vi "MNIST_weight print_sub.vi"(1 "최소값":dbl=-255.0, 2 "최대값":dbl=255.0, 3 "배열":dbl[][](array[numeric])=[[-5.0, -1.0, 4.0, -1.0, -5.0, -4.0, -5.0, -5.0, -5.0, -1.0, 4.0, -2.0, -5.0, -4.0, 4.0, 4.0, 5.0, 4.0, 4.0, 2.0, -3.0, -5.0, -1.0, 3.0, 5.0, 5.0, 0.0, 1.0], [-4.0, -5.0, 4.0, 2.0, 3.0, 5.0, -3.0, -5.0, -5.0, -5.0, -5.0, -5.0, -5.0, -5.0, -5.0, -5.0, -5.0, -5.0, -5.0, -5.0, -5.0, -5.0, -5.0, -5.0, -1.0, -5.0, 5.0, -3.0], [0.0, -5.0, -5.0, -5.0, -5.0, -5.0, -5.0, -5.0, -5.0, -5.0, -6.0, -6.0, -6.0, -6.0, -6.0, -6.0, -6.0, -7.0, -6.0, -6.0, -6.0, -6.0, -5.0, -5.0, 4.0, 4.0, -5.0, -2.0], [-2.0, -5.0, 2.0, -5.0, -5.0, -5.0, -5.0, -6.0, -6.0, -6.0, -7.0, -7.0, -7.0, -8.0, -10.0, -10.0, -7.0, -7.0, -9.0, -7.0, -10.0, -8.0, -7.0, -7.0, -6.0, -2.0, 0.0, 0.0], [-5.0, -5.0, 2.0, -5.0, -1.0, -5.0, -6.0, -7.0, -10.0, -15.0, -15.0, -14.0, -14.0, -12.0, -14.0, -26.0, -26.0, -18.0, -18.0, -22.0, -23.0, -19.0, -14.0, -9.0, -7.0, -5.0, -5.0, -5.0], [-5.0, 0.0, 2.0, -5.0, -5.0, -7.0, -7.0, -9.0, -14.0, -28.0, -32.0, -42.0, -44.0, -45.0, -53.0, -58.0, -56.0, -63.0, -53.0, -45.0, -47.0, -42.0, -29.0, -18.0, -10.0, -7.0, -5.0, -5.0], [5.0, -5.0, -5.0, -6.0, -8.0, -7.0, -10.0, -22.0, -30.0, -44.0, -37.0, -25.0, 7.0, 28.0, 51.0, 43.0, 22.0, -1.0, -16.0, -39.0, -51.0, -48.0, -35.0, -17.0, -9.0, -7.0, -6.0, -5.0], [1.0, -5.0, -7.0, -8.0, -8.0, -11.0, -17.0, -29.0, -37.0, -30.0, -3.0, 31.0, 72.0, 92.0, 96.0, 93.0, 86.0, 52.0, 27.0, -12.0, -39.0, -45.0, -29.0, -10.0, -9.0, -7.0, -7.0, -5.0], [-5.0, -6.0, -7.0, -8.0, -10.0, -16.0, -17.0, -23.0, -15.0, -9.0, 24.0, 66.0, 83.0, 55.0, 34.0, 22.0, 45.0, 38.0, 30.0, 5.0, -22.0, -34.0, -31.0, -20.0, -11.0, -8.0, -7.0, -5.0], [-5.0, -6.0, -7.0, -7.0, -14.0, -15.0, -10.0, -8.0, 6.0, 21.0, 62.0, 73.0, 34.0, 4.0, -19.0, -36.0, -5.0, 16.0, 29.0, 24.0, 2.0, -21.0, -31.0, -17.0, -12.0, -8.0, -7.0, -5.0], [-5.0, -6.0, -7.0, -7.0, -16.0, -7.0, 10.0, 21.0, 28.0, 41.0, 56.0, 38.0, 0.0, -25.0, -40.0, -19.0, 13.0, 34.0, 36.0, 35.0, 16.0, -14.0, -19.0, -12.0, -8.0, -7.0, -7.0, -5.0], [-5.0, -6.0, -7.0, -7.0, -11.0, 7.0, 15.0, 42.0, 53.0, 44.0, 35.0, 9.0, -43.0, -46.0, -33.0, -10.0, 35.0, 51.0, 58.0, 60.0, 27.0, 6.0, -14.0, -9.0, -7.0, -6.0, -6.0, -5.0], [-5.0, -6.0, -6.0, -5.0, 7.0, 14.0, 30.0, 59.0, 56.0, 33.0, 14.0, -17.0, -48.0, -42.0, -24.0, 9.0, 35.0, 47.0, 75.0, 74.0, 27.0, -1.0, -12.0, -10.0, -7.0, -7.0, -7.0, -5.0], [-5.0, -5.0, -6.0, -2.0, 7.0, 17.0, 37.0, 64.0, 65.0, 19.0, 10.0, -19.0, -40.0, -18.0, -8.0, 10.0, 44.0, 72.0, 71.0, 43.0, 8.0, -4.0, -17.0, -17.0, -9.0, -7.0, -6.0, -5.0], [-5.0, -5.0, -6.0, 4.0, 3.0, 8.0, 26.0, 58.0, 67.0, 24.0, 7.0, -4.0, -4.0, -10.0, -4.0, 25.0, 60.0, 89.0, 60.0, 5.0, -26.0, -29.0, -21.0, -20.0, -10.0, -6.0, -5.0, -4.0], [-5.0, 5.0, -7.0, -8.0, -5.0, -7.0, 12.0, 39.0, 60.0, 48.0, 45.0, 33.0, 23.0, 3.0, 14.0, 42.0, 75.0, 66.0, 21.0, -21.0, -41.0, -43.0, -25.0, -17.0, -10.0, -6.0, -5.0, -5.0], [-5.0, -5.0, -6.0, -9.0, -9.0, -18.0, -2.0, 18.0, 42.0, 46.0, 55.0, 42.0, 18.0, 7.0, 22.0, 51.0, 65.0, 55.0, -2.0, -25.0, -35.0, -44.0, -18.0, -15.0, -10.0, -7.0, -5.0, -5.0], [-4.0, -5.0, -5.0, -8.0, -15.0, -23.0, -12.0, 1.0, 18.0, 28.0, 44.0, 37.0, 22.0, 13.0, 25.0, 59.0, 58.0, 28.0, 7.0, -21.0, -46.0, -40.0, -24.0, -14.0, -9.0, -6.0, -5.0, -5.0], [5.0, -5.0, -5.0, -7.0, -13.0, -23.0, -25.0, -11.0, -8.0, -9.0, 9.0, 1.0, -1.0, 4.0, 17.0, 48.0, 50.0, 14.0, 4.0, -16.0, -38.0, -31.0, -22.0, -14.0, -8.0, -7.0, -6.0, -5.0], [3.0, -5.0, -7.0, -7.0, -10.0, -25.0, -41.0, -37.0, -28.0, -30.0, -29.0, -26.0, -24.0, -14.0, 2.0, 23.0, 24.0, -5.0, 1.0, -17.0, -29.0, -20.0, -17.0, -10.0, -7.0, -7.0, -5.0, -5.0], [-5.0, -5.0, -6.0, -7.0, -10.0, -18.0, -36.0, -45.0, -49.0, -54.0, -60.0, -53.0, -43.0, -29.0, -1.0, 3.0, 5.0, -15.0, -9.0, -11.0, -20.0, -14.0, -10.0, -10.0, 0.0, 2.0, -5.0, 0.0], [0.0, -5.0, -6.0, -7.0, -9.0, -14.0, -30.0, -42.0, -44.0, -50.0, -61.0, -56.0, -52.0, -42.0, -21.0, -22.0, -6.0, -16.0, -2.0, -3.0, -8.0, -11.0, -9.0, -6.0, 5.0, -2.0, -5.0, -3.0], [-2.0, -5.0, -7.0, -5.0, -7.0, -13.0, -23.0, -30.0, -39.0, -50.0, -49.0, -57.0, -56.0, -43.0, -34.0, -19.0, -11.0, -9.0, 13.0, 12.0, -2.0, 1.0, 8.0, 8.0, 2.0, -5.0, -6.0, 1.0], [3.0, 5.0, -6.0, -5.0, -7.0, -10.0, -14.0, -25.0, -28.0, -23.0, -24.0, -24.0, -26.0, -26.0, -17.0, -12.0, 3.0, 7.0, 30.0, 32.0, 12.0, 7.0, 9.0, 9.0, 6.0, -5.0, -5.0, -5.0], [5.0, 0.0, -5.0, -6.0, -7.0, -3.0, -6.0, -9.0, -3.0, 6.0, -1.0, 0.0, 11.0, 25.0, 34.0, 27.0, 24.0, 38.0, 53.0, 49.0, 20.0, 9.0, 9.0, 9.0, 0.0, -5.0, -5.0, 0.0], [3.0, 5.0, 5.0, -6.0, 4.0, 6.0, 7.0, 6.0, 13.0, 14.0, 15.0, 23.0, 36.0, 46.0, 41.0, 31.0, 35.0, 44.0, 57.0, 35.0, 15.0, 9.0, 7.0, 7.0, -1.0, -5.0, -5.0, -2.0], [-4.0, 5.0, -1.0, 5.0, 6.0, 7.0, 8.0, 7.0, 5.0, 2.0, 6.0, 9.0, 11.0, 16.0, 14.0, 7.0, 6.0, 6.0, 12.0, 12.0, 10.0, 7.0, 5.0, 5.0, 5.0, -5.0, 5.0, -5.0], [-2.0, 4.0, -5.0, 4.0, -5.0, -5.0, 4.0, 5.0, 5.0, 1.0, 0.0, 0.0, -5.0, -7.0, 1.0, -1.0, -8.0, -6.0, -5.0, -5.0, 5.0, -5.0, -5.0, -5.0, 5.0, -5.0, 5.0, -4.0], [-5.0, 0.0, 0.0, 0.0, 0.0, 0.0, 0.0, 0.0, 0.0, 0.0, 0.0, 0.0, 0.0, 0.0, 0.0, 0.0, 0.0, 0.0, 0.0, 0.0, 0.0, 0.0, 0.0, 0.0, 0.0, 0.0, 0.0, 0.0]]) -> (0 "MNIST_Input":dbl[][](graph)=[[-5.0, -1.0, 4.0, -1.0, -5.0, -4.0, -5.0, -5.0, -5.0, -1.0, 4.0, -2.0, -5.0, -4.0, 4.0, 4.0, 5.0, 4.0, 4.0, 2.0, -3.0, -5.0, -1.0, 3.0, 5.0, 5.0, 0.0, 1.0], [-4.0, -5.0, 4.0, 2.0, 3.0, 5.0, -3.0, -5.0, -5.0, -5.0, -5.0, -5.0, -5.0, -5.0, -5.0, -5.0, -5.0, -5.0, -5.0, -5.0, -5.0, -5.0, -5.0, -5.0, -1.0, -5.0, 5.0, -3.0], [0.0, -5.0, -5.0, -5.0, -5.0, -5.0, -5.0, -5.0, -5.0, -5.0, -6.0, -6.0, -6.0, -6.0, -6.0, -6.0, -6.0, -7.0, -6.0, -6.0, -6.0, -6.0, -5.0, -5.0, 4.0, 4.0, -5.0, -2.0], [-2.0, -5.0, 2.0, -5.0, -5.0, -5.0, -5.0, -6.0, -6.0, -6.0, -7.0, -7.0, -7.0, -8.0, -10.0, -10.0, -7.0, -7.0, -9.0, -7.0, -10.0, -8.0, -7.0, -7.0, -6.0, -2.0, 0.0, 0.0], [-5.0, -5.0, 2.0, -5.0, -1.0, -5.0, -6.0, -7.0, -10.0, -15.0, -15.0, -14.0, -14.0, -12.0, -14.0, -26.0, -26.0, -18.0, -18.0, -22.0, -23.0, -19.0, -14.0, -9.0, -7.0, -5.0, -5.0, -5.0], [-5.0, 0.0, 2.0, -5.0, -5.0, -7.0, -7.0, -9.0, -14.0, -28.0, -32.0, -42.0, -44.0, -45.0, -53.0, -58.0, -56.0, -63.0, -53.0, -45.0, -47.0, -42.0, -29.0, -18.0, -10.0, -7.0, -5.0, -5.0], [5.0, -5.0, -5.0, -6.0, -8.0, -7.0, -10.0, -22.0, -30.0, -44.0, -37.0, -25.0, 7.0, 28.0, 51.0, 43.0, 22.0, -1.0, -16.0, -39.0, -51.0, -48.0, -35.0, -17.0, -9.0, -7.0, -6.0, -5.0], [1.0, -5.0, -7.0, -8.0, -8.0, -11.0, -17.0, -29.0, -37.0, -30.0, -3.0, 31.0, 72.0, 92.0, 96.0, 93.0, 86.0, 52.0, 27.0, -12.0, -39.0, -45.0, -29.0, -10.0, -9.0, -7.0, -7.0, -5.0], [-5.0, -6.0, -7.0, -8.0, -10.0, -16.0, -17.0, -23.0, -15.0, -9.0, 24.0, 66.0, 83.0, 55.0, 34.0, 22.0, 45.0, 38.0, 30.0, 5.0, -22.0, -34.0, -31.0, -20.0, -11.0, -8.0, -7.0, -5.0], [-5.0, -6.0, -7.0, -7.0, -14.0, -15.0, -10.0, -8.0, 6.0, 21.0, 62.0, 73.0, 34.0, 4.0, -19.0, -36.0, -5.0, 16.0, 29.0, 24.0, 2.0, -21.0, -31.0, -17.0, -12.0, -8.0, -7.0, -5.0], [-5.0, -6.0, -7.0, -7.0, -16.0, -7.0, 10.0, 21.0, 28.0, 41.0, 56.0, 38.0, 0.0, -25.0, -40.0, -19.0, 13.0, 34.0, 36.0, 35.0, 16.0, -14.0, -19.0, -12.0, -8.0, -7.0, -7.0, -5.0], [-5.0, -6.0, -7.0, -7.0, -11.0, 7.0, 15.0, 42.0, 53.0, 44.0, 35.0, 9.0, -43.0, -46.0, -33.0, -10.0, 35.0, 51.0, 58.0, 60.0, 27.0, 6.0, -14.0, -9.0, -7.0, -6.0, -6.0, -5.0], [-5.0, -6.0, -6.0, -5.0, 7.0, 14.0, 30.0, 59.0, 56.0, 33.0, 14.0, -17.0, -48.0, -42.0, -24.0, 9.0, 35.0, 47.0, 75.0, 74.0, 27.0, -1.0, -12.0, -10.0, -7.0, -7.0, -7.0, -5.0], [-5.0, -5.0, -6.0, -2.0, 7.0, 17.0, 37.0, 64.0, 65.0, 19.0, 10.0, -19.0, -40.0, -18.0, -8.0, 10.0, 44.0, 72.0, 71.0, 43.0, 8.0, -4.0, -17.0, -17.0, -9.0, -7.0, -6.0, -5.0], [-5.0, -5.0, -6.0, 4.0, 3.0, 8.0, 26.0, 58.0, 67.0, 24.0, 7.0, -4.0, -4.0, -10.0, -4.0, 25.0, 60.0, 89.0, 60.0, 5.0, -26.0, -29.0, -21.0, -20.0, -10.0, -6.0, -5.0, -4.0], [-5.0, 5.0, -7.0, -8.0, -5.0, -7.0, 12.0, 39.0, 60.0, 48.0, 45.0, 33.0, 23.0, 3.0, 14.0, 42.0, 75.0, 66.0, 21.0, -21.0, -41.0, -43.0, -25.0, -17.0, -10.0, -6.0, -5.0, -5.0], [-5.0, -5.0, -6.0, -9.0, -9.0, -18.0, -2.0, 18.0, 42.0, 46.0, 55.0, 42.0, 18.0, 7.0, 22.0, 51.0, 65.0, 55.0, -2.0, -25.0, -35.0, -44.0, -18.0, -15.0, -10.0, -7.0, -5.0, -5.0], [-4.0, -5.0, -5.0, -8.0, -15.0, -23.0, -12.0, 1.0, 18.0, 28.0, 44.0, 37.0, 22.0, 13.0, 25.0, 59.0, 58.0, 28.0, 7.0, -21.0, -46.0, -40.0, -24.0, -14.0, -9.0, -6.0, -5.0, -5.0], [5.0, -5.0, -5.0, -7.0, -13.0, -23.0, -25.0, -11.0, -8.0, -9.0, 9.0, 1.0, -1.0, 4.0, 17.0, 48.0, 50.0, 14.0, 4.0, -16.0, -38.0, -31.0, -22.0, -14.0, -8.0, -7.0, -6.0, -5.0], [3.0, -5.0, -7.0, -7.0, -10.0, -25.0, -41.0, -37.0, -28.0, -30.0, -29.0, -26.0, -24.0, -14.0, 2.0, 23.0, 24.0, -5.0, 1.0, -17.0, -29.0, -20.0, -17.0, -10.0, -7.0, -7.0, -5.0, -5.0], [-5.0, -5.0, -6.0, -7.0, -10.0, -18.0, -36.0, -45.0, -49.0, -54.0, -60.0, -53.0, -43.0, -29.0, -1.0, 3.0, 5.0, -15.0, -9.0, -11.0, -20.0, -14.0, -10.0, -10.0, 0.0, 2.0, -5.0, 0.0], [0.0, -5.0, -6.0, -7.0, -9.0, -14.0, -30.0, -42.0, -44.0, -50.0, -61.0, -56.0, -52.0, -42.0, -21.0, -22.0, -6.0, -16.0, -2.0, -3.0, -8.0, -11.0, -9.0, -6.0, 5.0, -2.0, -5.0, -3.0], [-2.0, -5.0, -7.0, -5.0, -7.0, -13.0, -23.0, -30.0, -39.0, -50.0, -49.0, -57.0, -56.0, -43.0, -34.0, -19.0, -11.0, -9.0, 13.0, 12.0, -2.0, 1.0, 8.0, 8.0, 2.0, -5.0, -6.0, 1.0], [3.0, 5.0, -6.0, -5.0, -7.0, -10.0, -14.0, -25.0, -28.0, -23.0, -24.0, -24.0, -26.0, -26.0, -17.0, -12.0, 3.0, 7.0, 30.0, 32.0, 12.0, 7.0, 9.0, 9.0, 6.0, -5.0, -5.0, -5.0], [5.0, 0.0, -5.0, -6.0, -7.0, -3.0, -6.0, -9.0, -3.0, 6.0, -1.0, 0.0, 11.0, 25.0, 34.0, 27.0, 24.0, 38.0, 53.0, 49.0, 20.0, 9.0, 9.0, 9.0, 0.0, -5.0, -5.0, 0.0], [3.0, 5.0, 5.0, -6.0, 4.0, 6.0, 7.0, 6.0, 13.0, 14.0, 15.0, 23.0, 36.0, 46.0, 41.0, 31.0, 35.0, 44.0, 57.0, 35.0, 15.0, 9.0, 7.0, 7.0, -1.0, -5.0, -5.0, -2.0], [-4.0, 5.0, -1.0, 5.0, 6.0, 7.0, 8.0, 7.0, 5.0, 2.0, 6.0, 9.0, 11.0, 16.0, 14.0, 7.0, 6.0, 6.0, 12.0, 12.0, 10.0, 7.0, 5.0, 5.0, 5.0, -5.0, 5.0, -5.0], [-2.0, 4.0, -5.0, 4.0, -5.0, -5.0, 4.0, 5.0, 5.0, 1.0, 0.0, 0.0, -5.0, -7.0, 1.0, -1.0, -8.0, -6.0, -5.0, -5.0, 5.0, -5.0, -5.0, -5.0, 5.0, -5.0, 5.0, -4.0], [-5.0, 0.0, 0.0, 0.0, 0.0, 0.0, 0.0, 0.0, 0.0, 0.0, 0.0, 0.0, 0.0, 0.0, 0.0, 0.0, 0.0, 0.0, 0.0, 0.0, 0.0, 0.0, 0.0, 0.0, 0.0, 0.0, 0.0, 0.0]])   [LabVIEW 2021]
panel:
  in  "색선택 3":u32[](array[colorbox])=[16711680, 0, 255]
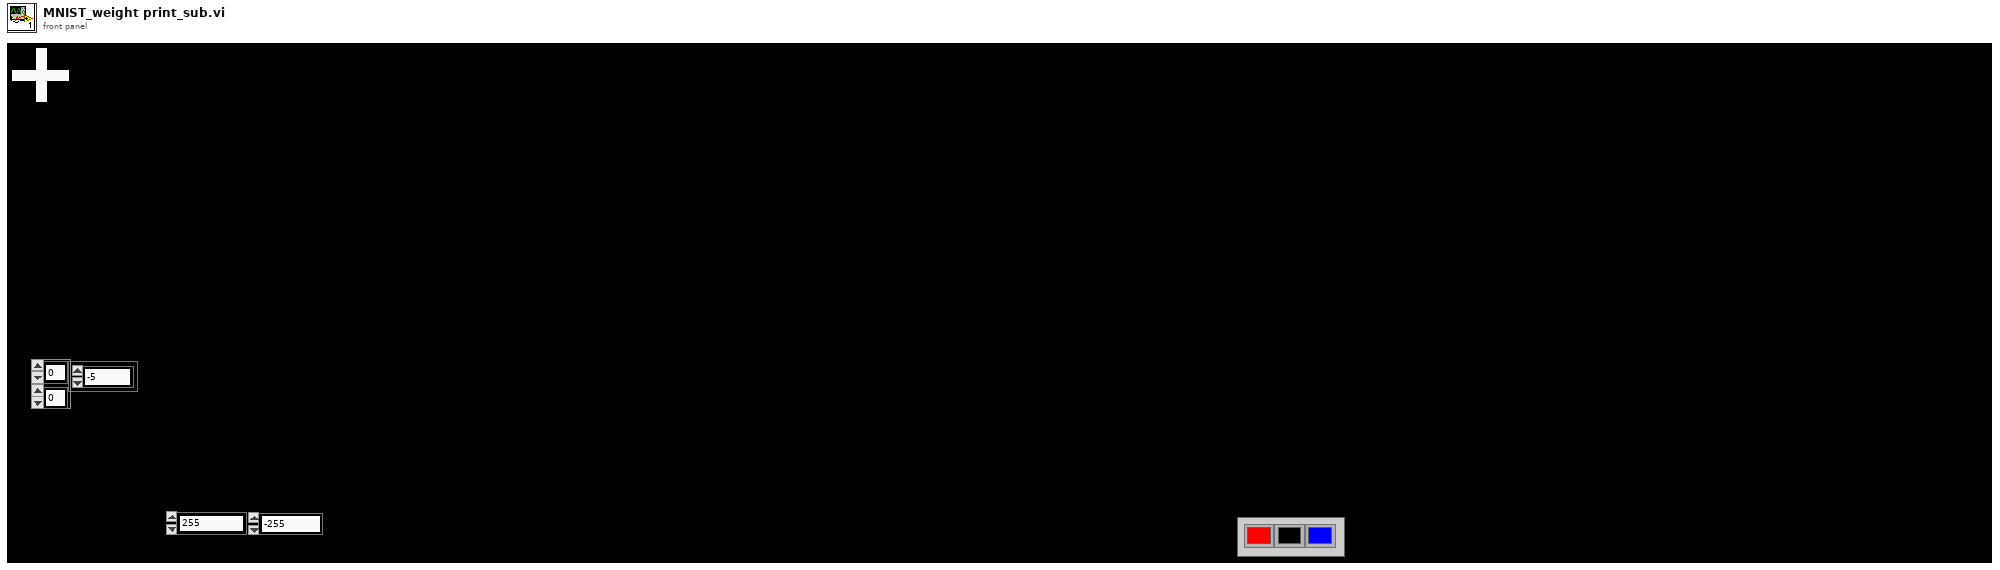
[diagram p1: front panel]
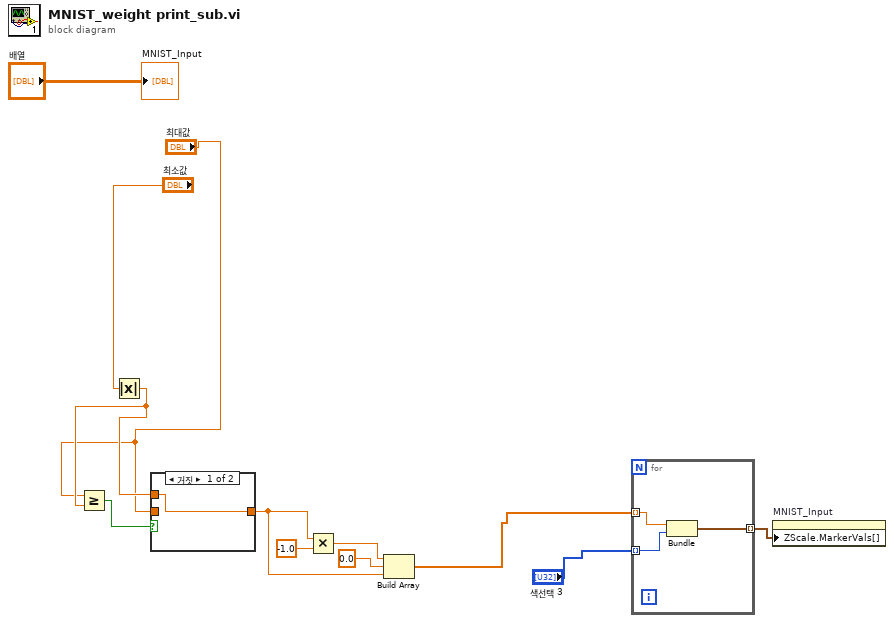
[diagram p0: block diagram]
diagram:
  n1 = Absolute Value(x="최소값") -> (abs(x)=w5:dbl)
  n2 = Greater Or Equal?(x="최대값", y=w5) -> (x >= y?=w11:bool)
  n3 = case shown="거짓" w11 {
    tunnel: "최대값" -> [_ w14]
    tunnel: [w13 w14] -> w7
    tunnel: w5 -> [w13 _]
    frame False {
    }
    frame True {
    }
  }
  n4 = Multiply(x=w7, y=-1.0) -> (x*y=w8:dbl)
  n5 = Build Array(w8, 0.0 ("원소"), w7) -> (w6:dbl[])
  n6 = for {
    tunnel: w6 -> [w17] mode=indexing
    tunnel: "색선택 3" -> [w16] mode=indexing
    tunnel: [w15] -> w2 mode=indexing
    n7 = Bundle("최대값"=w17, "색 상자"=w16) -> (w15:cluster{"최대값":dbl, "색 상자":u32})  [unwired: 1 in]
  }
  n8 = property on="MNIST_Input" class="IntGraph (엄격한)"("ZScale.MarkerVals[]"=w2) -> ()  [unwired: 2 in, 2 out]
  "MNIST_Input" <- "배열"
